vi "SoftIocPathName.vi"() -> (0 "pathName":string)   [LabVIEW 2018]
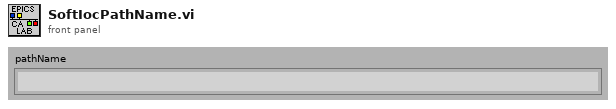
[diagram p1: front panel]
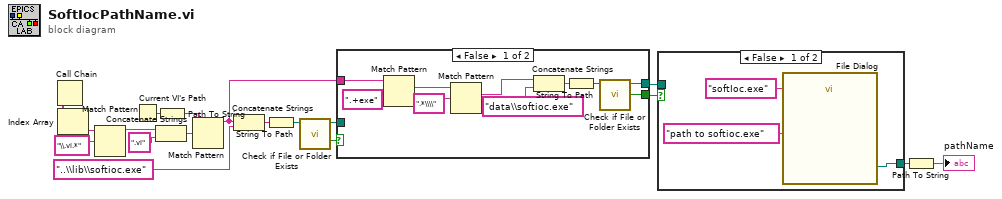
[diagram p0: block diagram]
diagram:
  n1 = Call Chain() -> (call chain=w17:string[])
  n2 = Index Array(array=w17) -> (element=w15:string)  [unwired: 1 in]
  n3 = Match Pattern(string=w15, regular expression="\\.vi.*") -> (before substring=w14:string)  [unwired: 4 out]
  n4 = Current VI's Path() -> (path=w18:path)
  n5 = Concatenate Strings(w14, ".vi" ("string")) -> (w12:string)
  n6 = Path To String(path=w18) -> (string=w11:string)
  n7 = Match Pattern(string=w11, regular expression=w12) -> (before substring=w5:string)  [unwired: 4 out]
  n8 = Concatenate Strings(w5, "..\\lib\\softioc.exe" ("string")) -> (w8:string)
  n9 = String To Path(string=w8) -> (path=w9:path)
  n10 = call <vilib>:"Check if File or Folder Exists.vi"("path"=w9) -> ("file or folder exists?"=w7:bool, "dup path"=w6:path)  [unwired: 1 in, 8 out]
  n11 = case shown="False" w7 {
    selector: w7 -> [_ w29]
    tunnel: w6 -> [_ w30]
    tunnel: w5 -> [w19 _]
    tunnel: [w25 w30] -> w4
    tunnel: [w24 w29] -> w3
    frame False {
      n12 = Match Pattern(string=w19, regular expression=".+exe" ("search string")) -> (match substring=w22:string)  [unwired: 1 in, 3 out]
      n13 = Match Pattern(string=w22, regular expression=".*\\\\") -> (match substring=w20:string)  [unwired: 1 in, 3 out]
      n14 = Concatenate Strings(w20, "data\\softioc.exe" ("string")) -> (w26:string)
      n15 = String To Path(string=w26) -> (path=w27:path)
      n16 = call <vilib>:"Check if File or Folder Exists.vi"("path"=w27) -> ("file or folder exists?"=w24:bool, "dup path"=w25:path)  [unwired: 1 in, 8 out]
    }
    frame True {
    }
  }
  n17 = case shown="False" w3 {
    tunnel: [w31 w34] -> w2
    tunnel: w4 -> [_ w34]
    frame False {
      n18 = call "File Dialog"("prompt"="path to softioc.exe" ("pattern label"), "default name"="softIoc.exe") -> ("selected path"=w31:path)  [unwired: 5 in, 8 out]
    }
    frame True {
    }
  }
  n19 = Path To String(path=w2) -> (string=→"pathName":string)
